vi "validate configuration.vi"(8 "error in":errorcluster, 11 "CVT configuration in":refnum<class "testmod configuration.lvclass">) -> (0 "error out":errorcluster, 3 "CVT configuration out":refnum<class "testmod configuration.lvclass">)   [LabVIEW 2013, in "testmod configuration.lvclass"]
doc: "This function performs validation of the configuration. This function should be safe to call at any point and should not rely on anything in the runtime environment."
uses:
  testmod configuration.lvclass
  <vilib>/NI/Tag Bus Module Framework/module configuration/TBM module configuration.lvclass
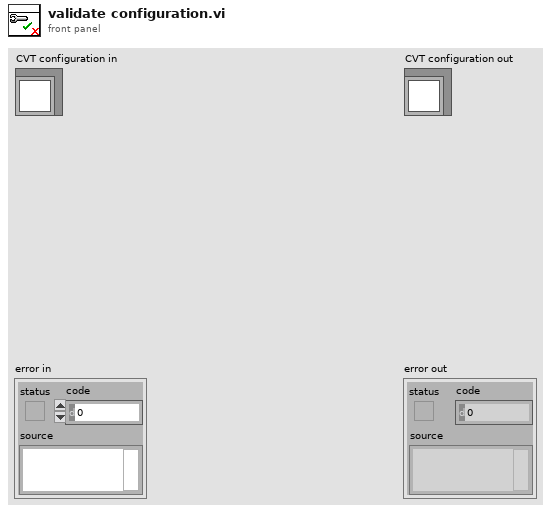
[diagram p1: front panel]
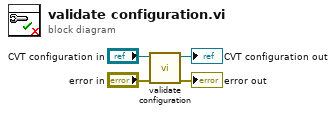
[diagram p0: block diagram]
diagram:
  n1 = call-parent "validate configuration.vi"("error in"="error in", "configuration in"="CVT configuration in") -> ("error out"=→"error out":errorcluster, "configuration out"=→"CVT configuration out":refnum<class "testmod configuration.lvclass">)  [unwired: 8 in]
